vi "ChangeMode.vi"(0 "reference in":refnum<class "Security.lvclass">, 2 "Security Mode":T1, 5 "Error In":errorcluster) -> (14 "reference out":refnum<class "Security.lvclass">, 19 "Error Out":errorcluster)   [LabVIEW 2024, in "Security.lvclass"]
uses:
  Security.lvclass
  Security.lvclass/Security.ctl
  Systems/SecuritySystem_class/Security Mode.ctl
  Systems/SecuritySystem_class/SecuritySystem.lvclass
panel:
  # "Connector Pane"
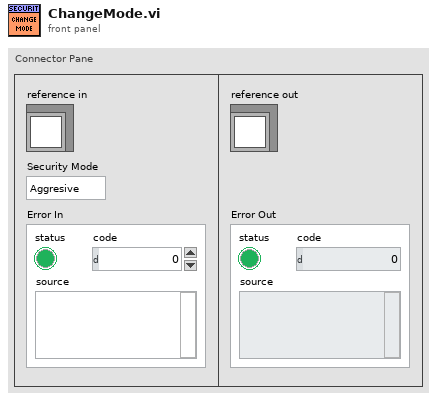
[diagram p1: front panel]
types:
  T1 = typedef "SecuritySystem.lvclass/Security Mode.ctl" = enum16{"Aggresive", "Defensive", "Balanced"}
  T2 = typedef "Security.lvclass/ObjectAttributes.ctl" = cluster{"State":bool, "Security Mode":T1}
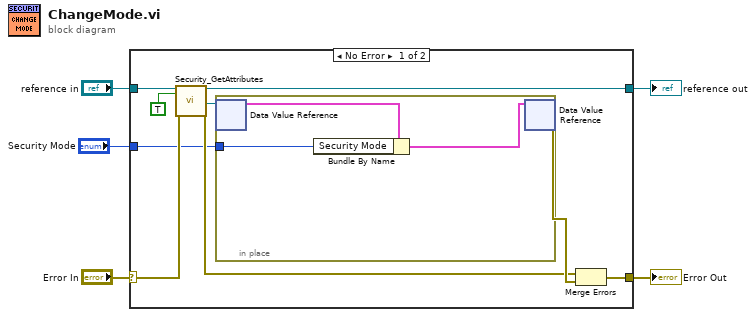
[diagram p0: block diagram]
diagram:
  n1 = case shown="No Error" "Error In" {
    selector: "Error In" -> [w13 w19]
    tunnel: [w7 w19] -> w4
    tunnel: [w12 w18] -> w2
    tunnel: "reference in" -> [w14 w18]
    tunnel: "Security Mode" -> [w6 _]
    frame No Error {
      n2 = call "Security_GetAttributes.vi"("reference in"=w14, "OnlyGetDvrReference(False)"=TRUE, "Error In"=w13) -> ("reference out"=w12:refnum<class "Security.lvclass">, "DataRef"=w9:refnum<data-value>, "Error Out"=w8:errorcluster)  [unwired: 13 in, 1 out]
      n3 = in-place {
        in-place-border: w6 -> [w15]
        n4 = in-place-dvr #1(w9) -> (w16:T2)  [unwired: 1 out]
        n5 = Bundle By Name(cluster=w16, "Security Mode"=w15) -> (w17:T2)
        n6 = in-place-dvr #1(w17) -> (w10:errorcluster)  [unwired: 1 out]
      }
      n7 = Merge Errors(w8, w10) -> (w7:errorcluster)
    }
    frame Error {
    }
  }
  "Error Out" <- w4
  "reference out" <- w2
